vi "Check - Folder Empty.vi"(11 "New QControl Info":refnum<data-value>) -> (0 "error out":errorcluster)   [LabVIEW 2019, in "New QControl Info.lvclass"]
doc: "<b> </b> <b> </b>\n©2016 Q Software Innovations, LLC (QSI)\nwritten by Quentin Alldredge\nproduced in LabVIEW 2015\n\nsupport@qsoftwareinnovations.com\nwww.qsoftwareinnovations.com\n\nAll rights reserved.\n\nRedistribution and use in source and binary forms, with or without modification, are permitted provided that the following conditions are met:\n\n * Redistributions of source code must retain the above copyright notice, this list of conditions and the following disclaimer.\n * Redistributions in binary form must reproduce the above copyright notice, this list of conditions and the following disclaimer in the documentation and/or other materials provided with the distribution.\n * Neither the name of Q Software Innovations, LLC. nor the names of its contributors may be used to endorse or promote products derived from this software without specific prior written permission.\n\nTHIS SOFTWARE IS PROVIDED BY THE COPYRIGHT HOLDERS AND CONTRIBUTORS \"AS IS\" AND ANY EXPRESS OR IMPLIED WARRANTIES, INCLUDING, BUT NOT LIMITED TO, THE IMPLIED WARRANTIES OF MERCHANTABILITY AND FITNESS FOR A PARTICULAR PURPOSE ARE DISCLAIMED. IN NO EVENT SHALL THE COPYRIGHT OWNER OR CONTRIBUTORS BE LIABLE FOR ANY DIRECT, INDIRECT, INCIDENTAL, SPECIAL, EXEMPLARY, OR CONSEQUENTIAL DAMAGES (INCLUDING, BUT NOT LIMITED TO, PROCUREMENT OF SUBSTITUTE GOODS OR SERVICES; LOSS OF USE, DATA, OR PROFITS; OR BUSINESS INTERRUPTION) HOWEVER CAUSED AND ON ANY THEORY OF LIABILITY, WHETHER IN CONTRACT, STRICT LIABILITY, OR TORT (INCLUDING NEGLIGENCE OR OTHERWISE) ARISING IN ANY WAY OUT OF THE USE OF THIS SOFTWARE, EVEN IF ADVISED OF THE POSSIBILITY OF SUCH DAMAGE."
uses:
  New QControl Info/New QControl Info.lvclass
  New QControl Info/New QControl Info.lvclass/New QControl Info.ctl
  New QControl Info/Read New Class Path.vi
  <vilib>/ErrorRing/Error Ring.xnode
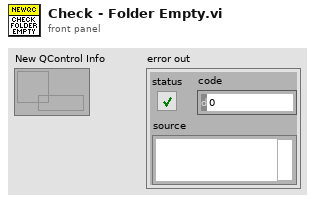
[diagram p1: front panel]
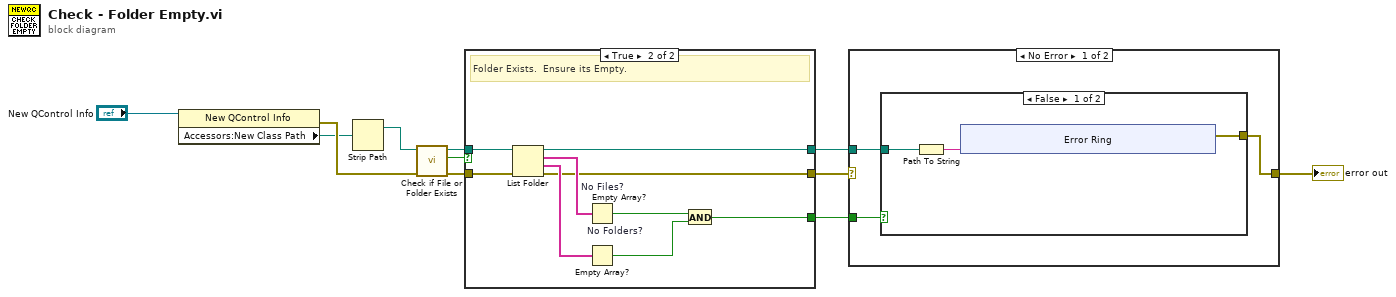
[diagram p0: block diagram]
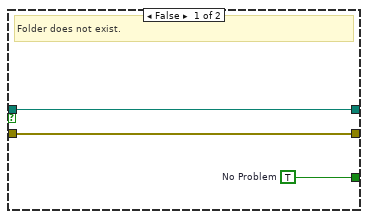
[diagram p2: hidden frame]
diagram:
  n1 = property class="New QControl Info"(reference="New QControl Info") -> (error out=w9:errorcluster, "Accessors:New Class Path"=w7:path)  [unwired: 1 in, 1 out]
  n2 = Strip Path(path=w7) -> (stripped path=w3:path)  [unwired: 1 out]
  n3 = call <vilib>:"Check if File or Folder Exists.vi"("error in (no error)"=w9, "path"=w3) -> ("error out"=w5:errorcluster, "file or folder exists?"=w8:bool, "dup path"=w6:path)  [unwired: 7 in]
  n4 = case shown="True" w8 {
    tunnel: w6 -> [w14 w23]
    tunnel: w5 -> [w12 w21]
    tunnel: [w13 w17] -> w4
    tunnel: [w14 w16] -> w2
    tunnel: [w12 w15] -> w1
    frame False {
      w13 = TRUE  # No Problem
      # "Folder does not exist."
    }
    frame True {
      # "Folder Exists.  Ensure its Empty."
      n5 = List Folder(path=w23, error in=w21) -> (path out=w16:path, filenames=w22:string[], folder names=w20:string[], error out=w15:errorcluster)  [unwired: 2 in]
      n6 = Empty Array? "No Files?"(array=w22) -> (empty?=w19:bool)
      n7 = Empty Array? "No Folders?"(array=w20) -> (empty?=w18:bool)
      n8 = And(x=w19, y=w18) -> (x .and. y?=w17:bool)
    }
  }
  n9 = case shown="No Error" w1 {
    selector: w1 -> [_ w35]
    tunnel: w4 -> [w26 _]
    tunnel: [w25 w35] -> w11
    tunnel: w2 -> [w24 _]
    frame No Error {
      n10 = case shown="False" w26 {
        tunnel: w24 -> [w29 _]
        tunnel: [w27 _] -> w25
        frame False {
          n11 = Path To String(path=w29) -> (string=w28:string)
          n12 = xnode "Error Ring"("parameter 0"=w28) -> ("error out"=w27:errorcluster)
        }
        frame True {
        }
      }
    }
    frame Error {
    }
  }
  "error out" <- w11
